vi "GetTemplatePaths.vi"(10 "Diameters":dbl[](array[numeric]), 11 "Folder":path) -> (1 "Templates 2D":path[][](array[path]), 2 "TemplateSources":path[](array[path]), 3 "Masks":path[](array[path]), 4 "Templates":path[](array[path]))   [LabVIEW 2015]
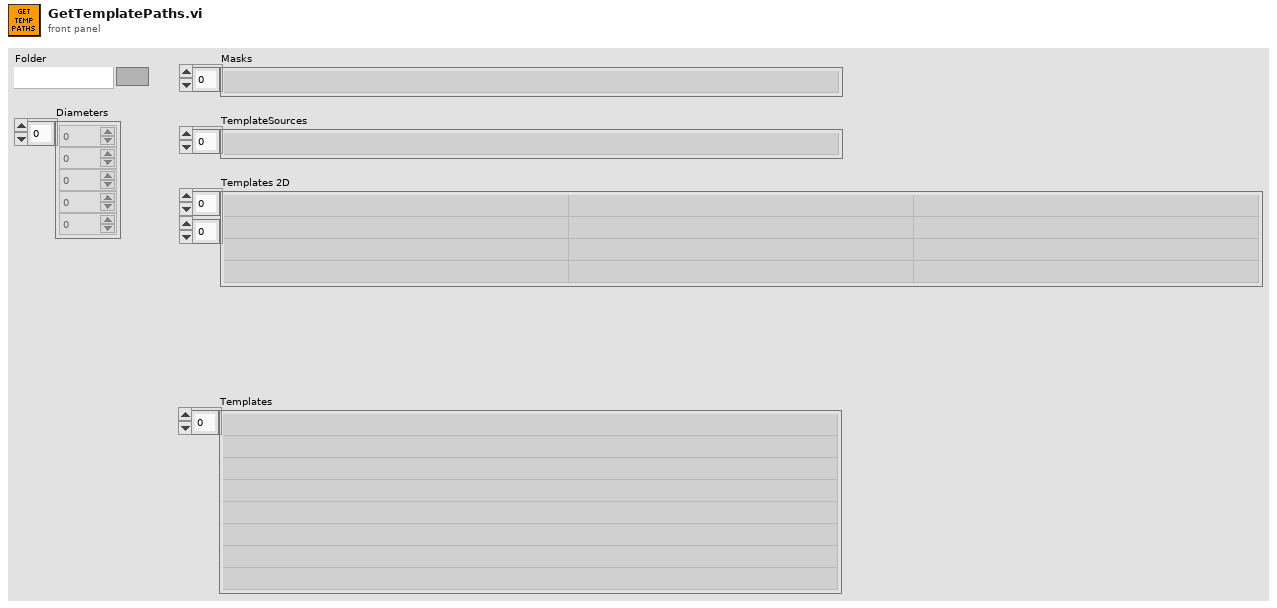
[diagram p1: front panel]
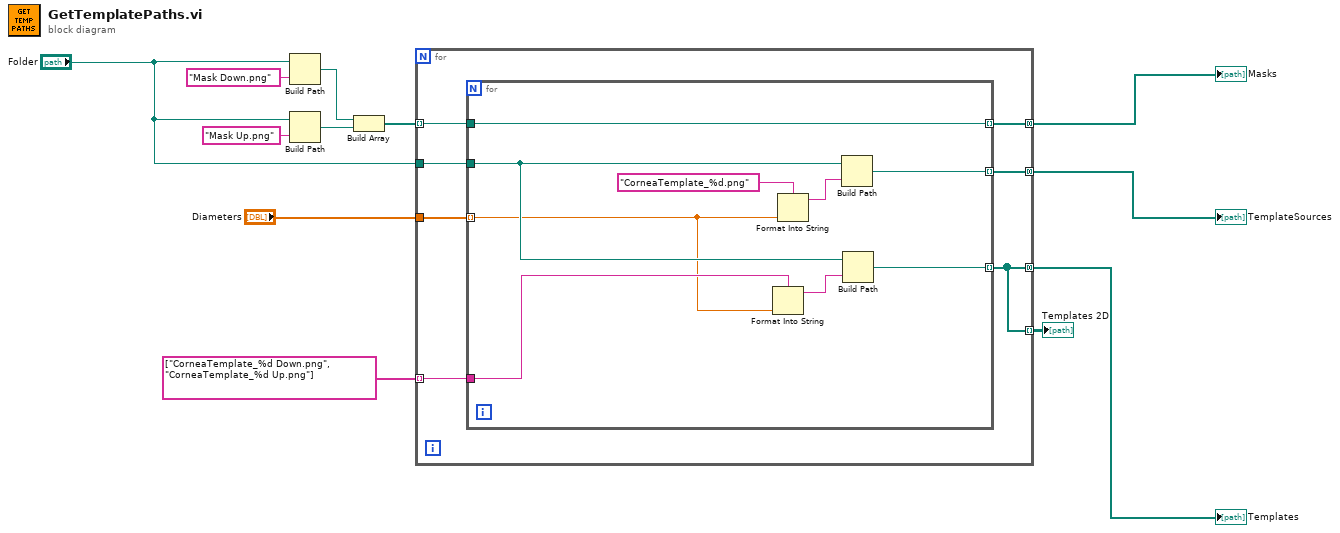
[diagram p0: block diagram]
diagram:
  n1 = Build Path(base path="Folder", name or relative path="Mask Down.png") -> (appended path=w3:path)
  n2 = Build Path(base path="Folder", name or relative path="Mask Up.png") -> (appended path=w4:path)
  n3 = Build Array(w3, w4) -> (w5:path[])
  n4 = for {
    tunnel: w5 -> [w17] mode=indexing
    tunnel: "Folder" -> [w19]
    tunnel: "Diameters" -> [w18]
    tunnel: [w16] -> w9 mode=concatenating
    tunnel: [w15] -> w10 mode=concatenating
    tunnel: string[] ["CorneaTemplate_%d Down.png", "CorneaTemplate_%d Up.png"] -> [w14] mode=indexing
    tunnel: [w13] -> w11 mode=concatenating
    tunnel: [w13] -> w12 mode=indexing
    n5 = for {
      tunnel: w19 -> [w25]
      tunnel: w18 -> [w20] mode=indexing
      tunnel: w17 -> [w24]
      tunnel: [w24] -> w16 mode=indexing
      tunnel: [w23] -> w15 mode=indexing
      tunnel: w14 -> [w22]
      tunnel: [w21] -> w13 mode=indexing
      n6 = Format Into String(format string=w22, w20) -> (resulting string=w28:string)  [unwired: 2 in, 1 out]
      n7 = Format Into String(format string="CorneaTemplate_%d.png" ("name or relative path"), w20) -> (resulting string=w27:string)  [unwired: 2 in, 1 out]
      n8 = Build Path(base path=w25, name or relative path=w27) -> (appended path=w23:path)
      n9 = Build Path(base path=w25, name or relative path=w28) -> (appended path=w21:path)
    }
  }
  "Templates 2D" <- w12
  "Templates" <- w11
  "TemplateSources" <- w10
  "Masks" <- w9
